vi "Read_Data_file.vi"(0 "Results file":path, 1 "Read Channel Names only":bool, 3 "Add Extra Channels?":bool, 5 "Template File":path, 8 "Desired File Types":T1) -> (10 "Row numbers":i32[](array[numeric]), 11 "Template File Out":path, 12 "Filetype":string, 13 "EOF?":bool, 14 "Results file Out":path, 15 "String Before":string, 16 "Ch names Out":string[](array[string]), 17 "Channel Values Out":string[][](array[string]), 18 "String After":string, 19 "mark after read (chars.)":i32)   [LabVIEW 2010]
uses:
  Data_File_Type.ctl
  Results_plotter_Global.vi
  Globals/Meas_global.vi
panel:
  out "Case":string
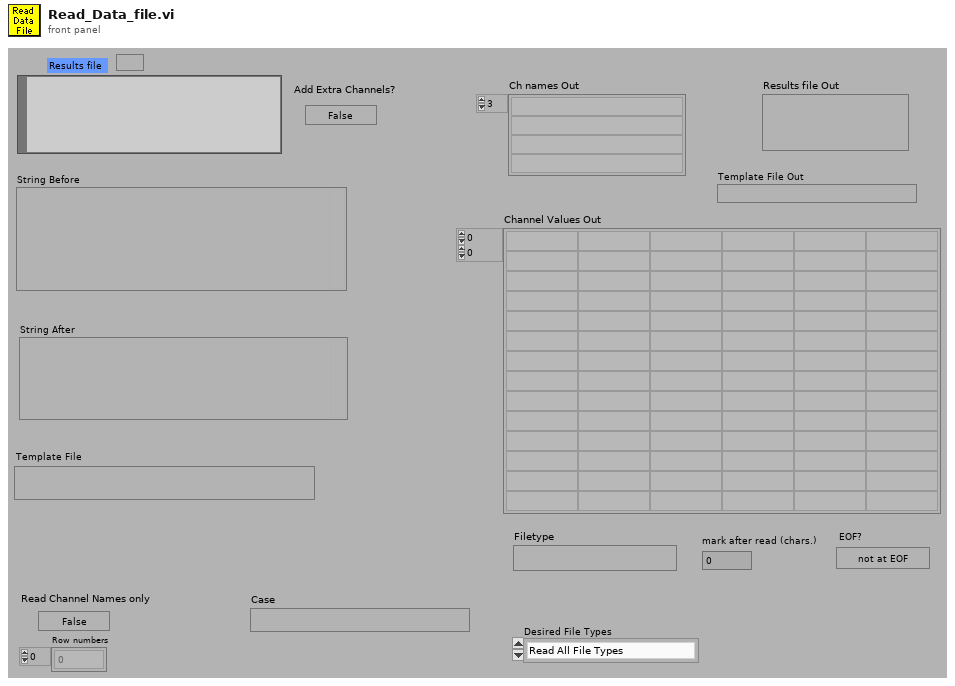
[diagram p1: front panel]
types:
  T1 = typedef "Data_File_Type.ctl" = enum16{"Read All File Types", "Results Files Only", "Raw Data Files Only", "Calibration Files Only", "Gas Desk Files Only", "Old Results Files Only", "Tabulated Data Files Only"}
  T2 = enum32{"existing file", "new file", "new or existing file", "existing dir", "new dir", "new or existing dir", "existing file (use LLBs)", "new file (use LLBs)", "new or existing file (use LLBs)", "new or existing file or directory (use LLBs)"}
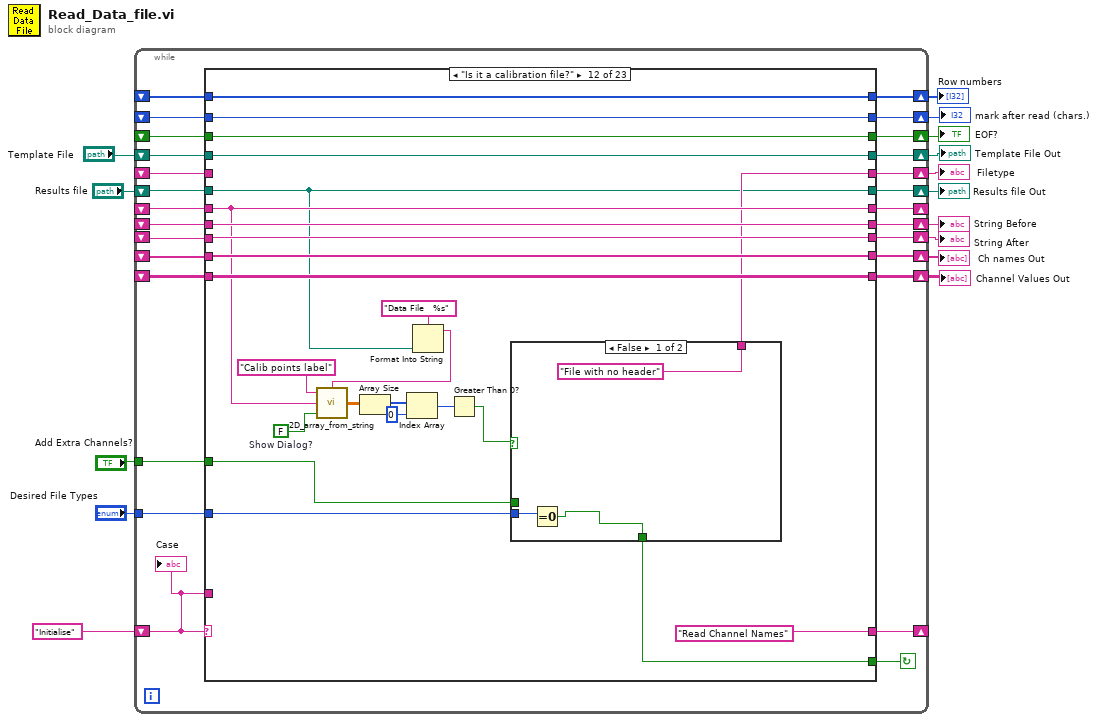
[diagram p0: block diagram]
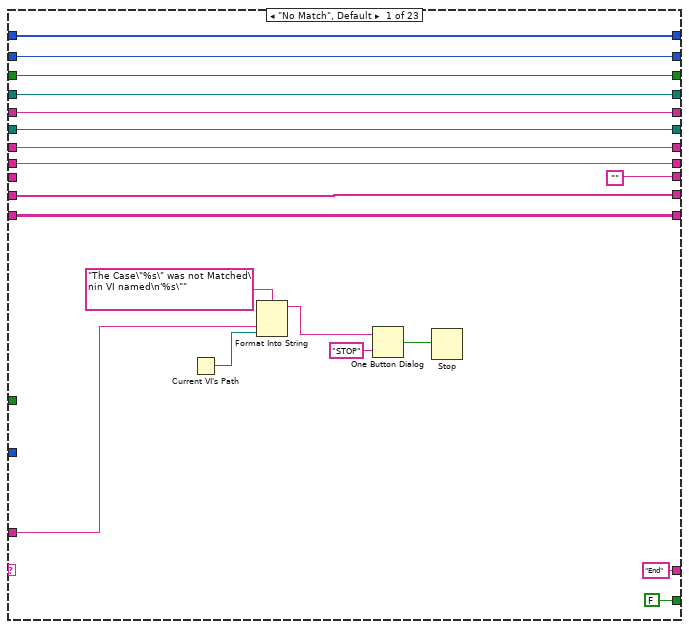
[diagram p2: hidden frame]
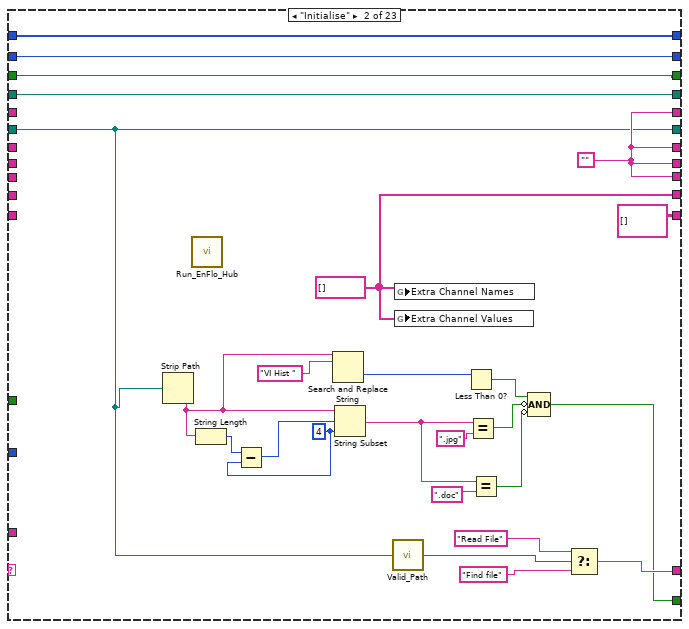
[diagram p3: hidden frame]
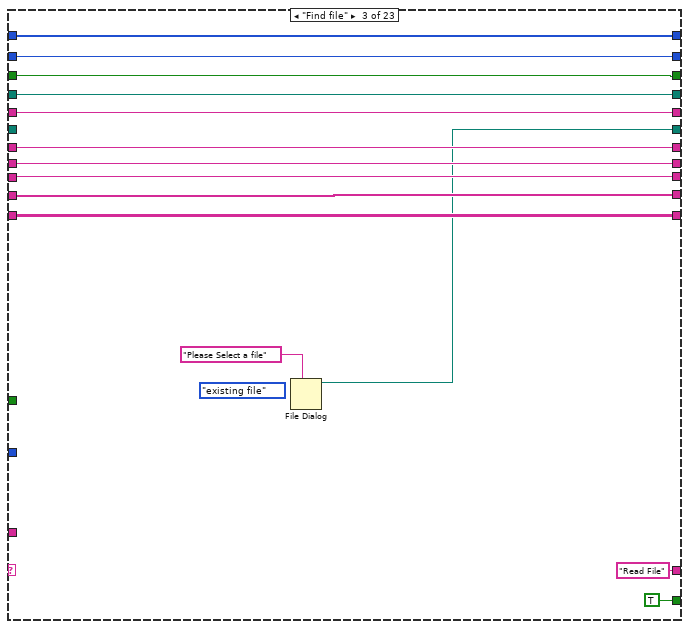
[diagram p4: hidden frame]
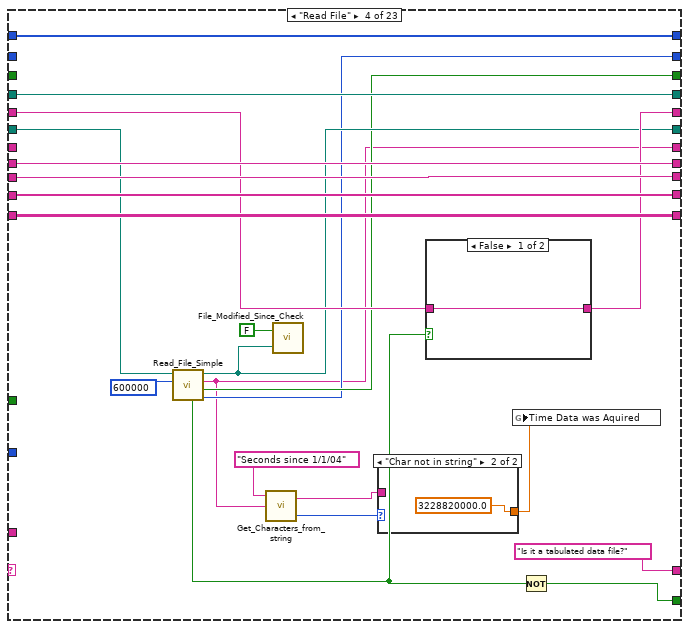
[diagram p5: hidden frame]
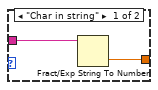
[diagram p6: hidden frame]
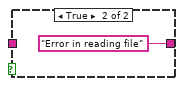
[diagram p7: hidden frame]
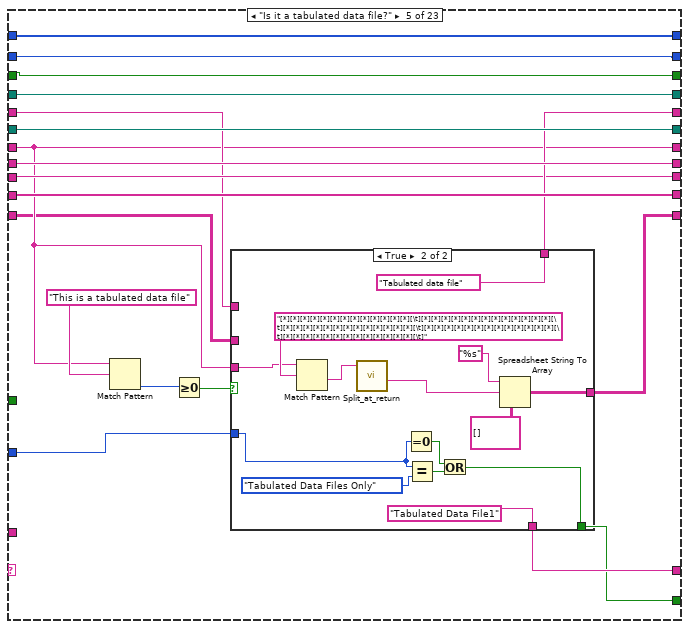
[diagram p8: hidden frame]
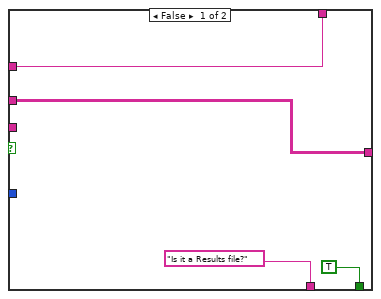
[diagram p9: hidden frame]
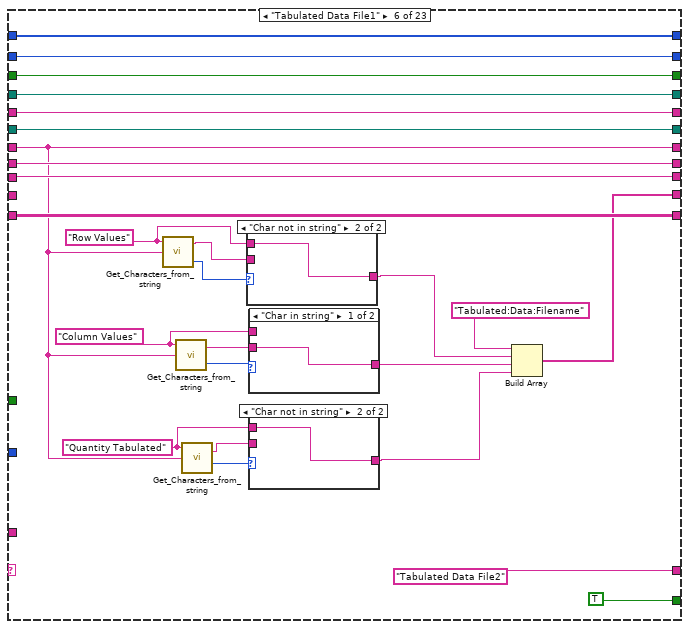
[diagram p10: hidden frame]
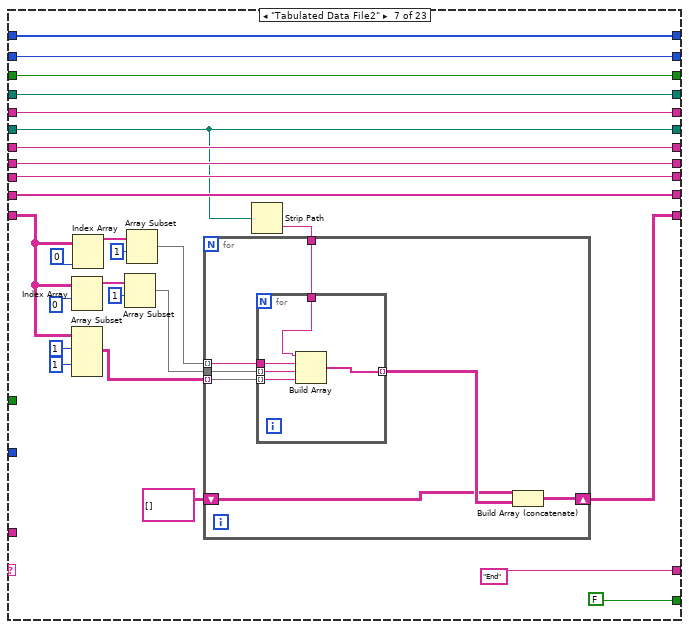
[diagram p14: hidden frame]
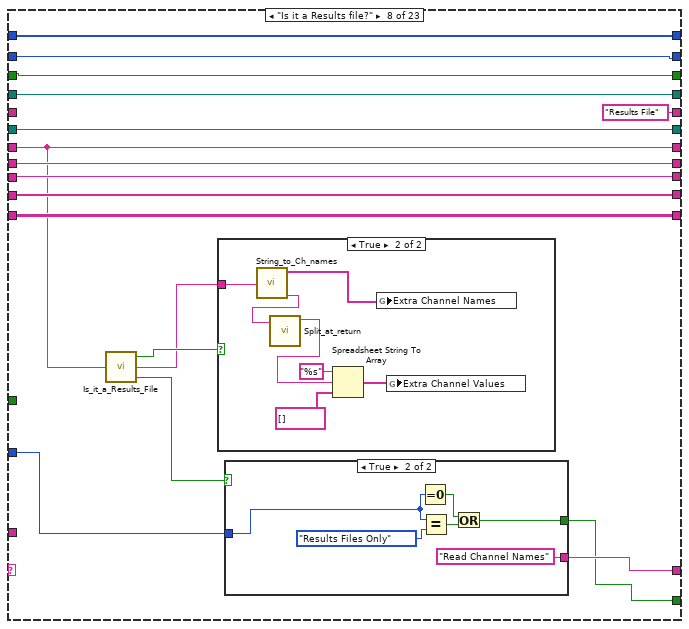
[diagram p15: hidden frame]
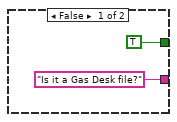
[diagram p16: hidden frame]
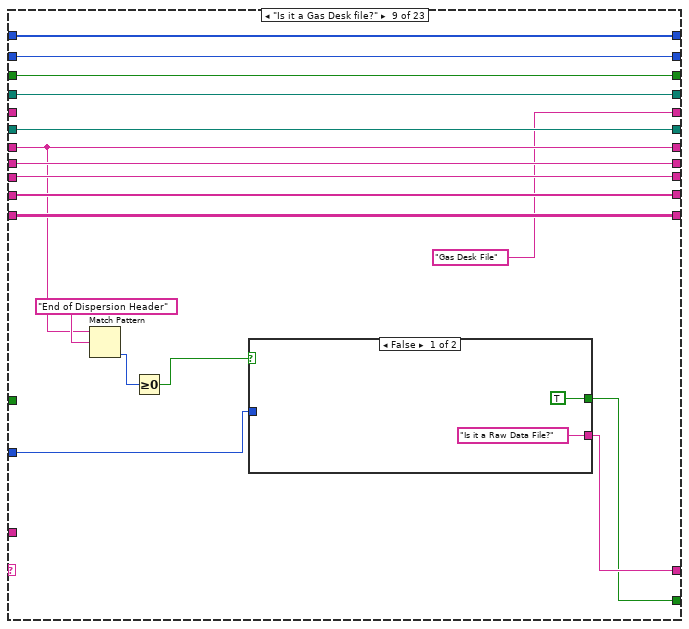
[diagram p18: hidden frame]
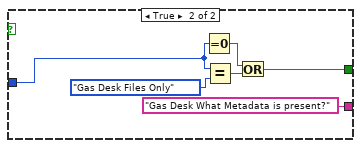
[diagram p19: hidden frame]
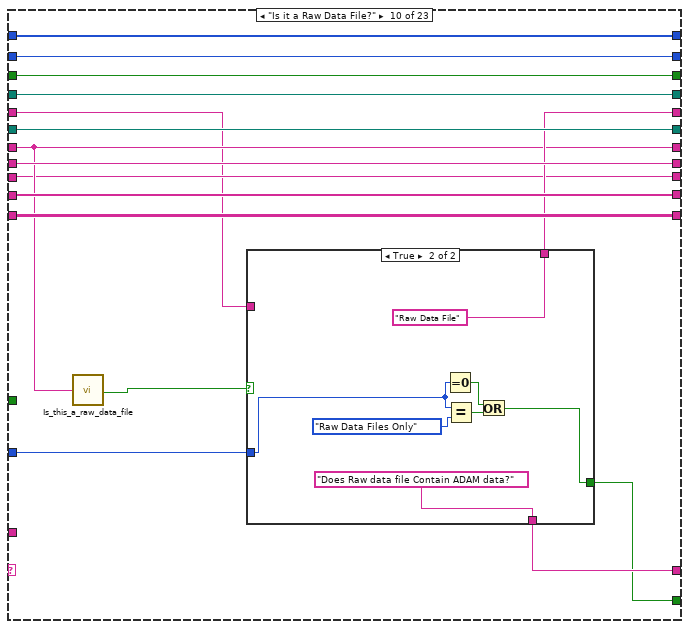
[diagram p20: hidden frame]
diagram:
  n1 = while {
    tunnel: "Add Extra Channels?" -> [w25]
    shift-left: _ -> [w29]
    shift-right: [w28] -> w14
    shift-left: "Results file" -> [w31]
    shift-right: [w30] -> w12
    shift-left: _ -> [w33]
    shift-right: [w32] -> w7
    shift-left: _ -> [w26]
    shift-right: [w34] -> w9
    shift-left: _ -> [w35]
    shift-right: [w36] -> _
    shift-left: "Initialise" -> [w39]
    shift-right: [w37] -> _
    shift-left: _ -> [w27]
    shift-right: [w41] -> w10
    shift-left: _ -> [w38]
    shift-right: [w42] -> w11
    shift-right: [w24] -> w6
    shift-left: "Template File" -> [w23]
    shift-right: [w21] -> w4
    shift-left: _ -> [w22]
    shift-right: [w20] -> w3
    shift-left: _ -> [w19]
    shift-right: [w17] -> w2
    shift-left: _ -> [w18]
    tunnel: "Desired File Types" -> [w16]
    stop <- w40 continue-if-true
    n2 = case shown="\"Is it a calibration file?\"" w39 {
      tunnel: [w54 w85 w99 w121 w146 w172 w223 w252 w284 w308 w336 w370 w404 w425 w464 w492 w505 w567 w590 w626 w652 w684 w703] -> w42
      tunnel: [w53 string[][] [] ("Channel Values") w98 w120 w135 w190 w212 w251 w283 w307 w335 w369 w403 w424 w463 w491 w513 w573 w615 w625 w647 w674 w699] -> w41
      tunnel: [FALSE ("Results File?") w74 TRUE ("Results File?") w117 w128 TRUE ("Results File?") FALSE ("Results File?") w243 w268 w294 w320 w356 w396 TRUE ("Results File?") TRUE ("Results File?") TRUE ("Results File?") w499 TRUE ("Results File?") TRUE ("Results File?") FALSE ("Results File?") TRUE ("Results File?") w678 FALSE ("Results File?")] -> w40
      tunnel: w39 -> [w56 _ _ _ _ _ _ _ _ _ _ _ _ _ _ _ _ _ _ _ _ _ _]
      tunnel: w38 -> [w54 _ w99 w121 w146 _ w223 w252 w284 w308 w336 w370 w404 w425 w464 w492 _ w567 w591 w630 w652 w684 w706]
      tunnel: ["End" w86 "Read File" "Is it a tabulated data file?" w142 "Tabulated Data File2" ("f") "End" ("f") w250 w269 w303 w331 "Read Channel Names" ("f") "Read Channel Names" ("f") w410 "Read Channel Names" ("f") "Read Channel Names" ("f") w503 "Does template file exist?" ("f") w610 "End" ("f") "Delete First Row?" ("f") "Add Extra Channels of data" ("f") "End" ("f")] -> w37
      tunnel: [w51 w83 w96 w103 w136 w183 w219 w245 w277 w301 w326 w365 w392 w412 w442 w475 w506 w568 w614 w631 w645 w686 w708] -> w36
      tunnel: w35 -> [w51 _ w96 _ w136 w183 w219 w245 w277 w301 w326 w365 w399 w411 w442 w475 w508 w568 w614 w631 w645 w686 w708]
      tunnel: [w50 w83 w95 w119 w144 w188 w222 w246 w280 w305 w333 w368 w401 w421 w460 w489 w507 w565 w613 w634 w651 w689 w712] -> w34
      tunnel: w33 -> [_ _ w94 w118 w141 w186 w220 w248 w281 w300 w330 w367 _ w422 w461 w490 w512 w572 w612 w633 w650 w688 w711]
      tunnel: ["" w83 w94 w118 w141 w186 w220 w248 w281 w300 w330 w367 w389 w422 w461 w490 w512 w572 w612 w633 w650 w688 w711] -> w32
      tunnel: w31 -> [w49 w67 _ w114 w145 w189 w202 w249 w282 w306 w334 w348 w402 w423 w462 w469 w511 w571 w608 w629 w644 w685 w707]
      tunnel: [w49 w67 w93 w110 w145 w189 w202 w249 w282 w306 w334 w348 w402 w423 w462 w469 w511 w571 w608 w629 w644 w685 w707] -> w30
      tunnel: w29 -> [w47 _ w91 w115 w140 w185 w218 _ _ w299 w329 _ w395 w409 w458 w487 w510 w570 w611 w628 w641 w683 w710]
      tunnel: [w47 w83 w91 w116 w143 w185 w218 "Results File" "Gas Desk File" w304 w332 w355 w395 w409 w458 w487 w510 w570 w611 w628 w641 w683 w710] -> w28
      tunnel: w27 -> [w53 _ w98 w120 w134 w190 w211 w251 w283 w307 w335 w369 w403 w424 w463 w491 w513 w573 w615 _ _ w682 w701]
      tunnel: w26 -> [w50 _ w95 w119 w144 w188 w222 w246 w280 w305 w333 w368 w401 w421 w460 w489 _ w565 w613 w634 w651 w689 w712]
      tunnel: w25 -> [_ _ _ _ _ _ _ _ _ _ _ w357 _ _ _ _ _ _ _ _ _ w669 _]
      tunnel: [w46 w73 w90 w109 w133 w168 w200 w241 w275 w298 w324 w354 w386 w408 w440 w468 w501 w563 w593 w624 w640 w677 w698] -> w24
      tunnel: w23 -> [w46 w73 w90 w109 w133 w168 w200 w241 w275 w298 w324 w354 w386 w408 w440 w468 w501 w563 w593 w623 w640 w677 w698]
      tunnel: w22 -> [w44 w71 w88 _ w131 w166 w198 w239 w273 w296 w322 w352 w384 w406 w438 w466 w500 w562 w602 w622 w639 w675 w696]
      tunnel: [w44 w71 w88 w108 w131 w166 w198 w239 w273 w296 w322 w352 w384 w406 w438 w466 w500 w562 w602 w622 w638 w675 w696] -> w21
      tunnel: [w45 w72 w89 w107 w132 w167 w199 w240 w274 w297 w323 w353 w385 w407 w439 w467 w496 w561 w601 w621 w637 w676 w697] -> w20
      tunnel: w19 -> [w45 w72 w89 _ w132 w167 w199 w240 w274 w297 w323 w353 w385 w407 w439 w467 w497 w561 w601 w621 w637 w676 w697]
      tunnel: [w43 w70 w87 w106 w130 w165 w197 w238 w272 w295 w321 w351 w383 w405 w437 w465 w493 w560 w600 w620 w636 w670 w695] -> w17
      tunnel: w18 -> [w43 w70 w87 w106 w130 w165 w197 w238 w272 w295 w321 w351 w383 w405 w437 w465 w493 w560 w600 _ w636 _ w695]
      tunnel: w16 -> [_ _ _ _ w129 _ _ w236 w271 w293 w319 w350 _ _ _ _ _ _ _ _ _ _ _]
      frame "No Match", Default {
        n3 = Current VI's Path() -> (path=w57:path)
        n4 = Format Into String(format string="The Case\"%s\" was not Matched\nin VI named\n'%s\"" ("Format String"), w56, w57) -> (resulting string=w60:string)  [unwired: 2 in, 1 out]
        n5 = One Button Dialog(message=w60, button name ("OK")="STOP") -> (true=w58:bool)
        n6 = Stop(stop? (T)=w58) -> ()
      }
      frame "Initialise" {
        w81 = 4 ("length (rest)")
        w83 = ""
        w85 = string[] [] ("Extra Channel Names")
        n7 = Strip Path(path=w67) -> (name=w79:string)  [unwired: 1 out]
        n8 = call "Run_EnFlo_Hub.vi"() -> ()  [unwired: 8 out]
        n9 = String Length(string=w79) -> (length=w82:i32)
        n10 = Subtract(x=w82, y=w81) -> (x-y=w80:i32)
        n11 = Search and Replace String(input string=w79, search string="VI Hist ") -> (offset past replacement=w77:i32)  [unwired: 1 in, 8 out]
        n12 = String Subset(string=w79, offset (0)=w80, length (rest)=w81) -> (substring=w64:string)
        n13 = call "Valid_Path.vi"("Filename"=w67) -> ("Valid Path?"=w66:bool)
        n14 = global write "Results_plotter_Global.vi" "Extra Channel Names"(w85) -> ()
        n15 = global write "Results_plotter_Global.vi" "Extra Channel Values"(w85) -> ()
        n16 = Less Than 0?(x=w77) -> (x < 0?=w75:bool)
        n17 = Equal?(x=w64, y=".jpg") -> (x = y?=w76:bool)
        n18 = Equal?(x=w64, y=".doc") -> (x = y?=w63:bool)
        n19 = Compound Arithmetic op=AND(w75, invert w76, invert w63) -> (w74:bool)
        n20 = Select(t="Read File", s=w66, f="Find file") -> (s? t:f=w86:string)
      }
      frame "Find file" {
        (unwired) T2."existing file" ("select mode (2)")
        n21 = File Dialog(7:"Please Select a file" ("prompt")) -> (3:w93:path)  [unwired: 1 in, 8 out]
      }
      frame "Read File" {
        n22 = call "Read_File_Simple.vi"("Filename"=w114, "number of characters (all:-1)"=600000 ("count")) -> ("Error?"=w112:bool, "Filename Out"=w110:path, "string"=w103:string, "EOF?"=w108:bool, "mark after read (chars.)"=w107:i32)  [unwired: 1 in, 3 out]
        n23 = call "Get_Characters_from_string.vi"("Input string"=w103, "Variable name"="Seconds since 1/1/04") -> ("Status"=w101:enum16{"Char in string", "Char not in string"}, "Value"=w104:string)  [unwired: 1 in]
        n24 = call "File_Modified_Since_Check.vi"("Pathname"=w110, "Just Modified?"=FALSE) -> ()  [unwired: 1 out]
        n25 = case shown="\"Char not in string\"" w101 {
          tunnel: w104 -> [w124 _]
          tunnel: [w123 3228820000.0 ("y")] -> w102
          frame "Char in string" {
            n26 = Fract/Exp String To Number(string=w124) -> (number=w123:dbl)  [unwired: 4 out]
          }
          frame "Char not in string" {
          }
        }
        n27 = case shown="False" w112 {
          tunnel: [w126 "Error in reading file"] -> w116
          tunnel: w115 -> [w126 _]
          frame False {
          }
          frame True {
          }
        }
        n28 = global write "Meas_global.vi" "Time Data was Aquired"(w102) -> ()
        n29 = Not(x=w112) -> (.not. x?=w117:bool)
      }
      frame "Is it a tabulated data file?" {
        n30 = Match Pattern(string=w136, regular expression="This is a tabulated data file") -> (offset past match=w139:i32)  [unwired: 4 out]
        n31 = Greater Or Equal To 0?(x=w139) -> (x >= 0?=w138:bool)
        n32 = case shown="True" w138 {
          tunnel: [w150 "Tabulated data file"] -> w143
          tunnel: ["Is it a Results file?" "Tabulated Data File1" ("f")] -> w142
          tunnel: w140 -> [w150 _]
          tunnel: w136 -> [_ w161]
          tunnel: [w149 w158] -> w135
          tunnel: w134 -> [w149 _]
          tunnel: w129 -> [_ w154]
          tunnel: [TRUE ("Results File?") w151] -> w128
          frame False {
          }
          frame True {
            n33 = Match Pattern(string=w161, regular expression="[*][*][*][*][*][*][*][*][*][*][*][*][*][\t][*][*][*][*][*][*][*][*][*][*][*][*][*][\t][*][*][*][*][*][*][*][*][*][*][*][*][*][\t][*][*][*][*][*][*][*][*][*][*][*][*][*][\t][*][*][*][*][*][*][*][*][*][*][*][*][*][\t]" ("String")) -> (after substring=w157:string)  [unwired: 4 out]
            n34 = call "Split_at_return.vi"("String"=w157) -> ("after substring"=w156:string)  [unwired: 1 in, 3 out]
            n35 = Equal To 0?(x=w154) -> (x = 0?=w152:bool)
            n36 = Equal?(x=w154, y=Data_File_Type."Tabulated Data Files Only" ("Desired File Types")) -> (x = y?=w153:bool)
            n37 = Or(x=w152, y=w153) -> (x .or. y?=w151:bool)
            n38 = Spreadsheet String To Array(format string="%s", spreadsheet string=w156, array type (2D Dbl)=string[][] [] ("Channel Values")) -> (array=w158:string[][])  [unwired: 1 out]
          }
        }
      }
      frame "Tabulated Data File1" {
        w171 = "Row Values" ("Variable name")
        w170 = "Column Values" ("Variable name")
        w177 = "Quantity Tabulated" ("Variable name")
        n39 = call "Get_Characters_from_string.vi"("Input string"=w183, "Variable name"=w171) -> ("Status"=w175:enum16{"Char in string", "Char not in string"}, "Value"=w176:string)  [unwired: 1 in]
        n40 = call "Get_Characters_from_string.vi"("Input string"=w183, "Variable name"=w170) -> ("Status"=w182:enum16{"Char in string", "Char not in string"}, "Value"=w181:string)  [unwired: 1 in]
        n41 = call "Get_Characters_from_string.vi"("Input string"=w183, "Variable name"=w177) -> ("Status"=w179:enum16{"Char in string", "Char not in string"}, "Value"=w178:string)  [unwired: 1 in]
        n42 = case shown="\"Char not in string\"" w175 {
          tunnel: w176 -> [w193 _]
          tunnel: [w193 w194] -> w174
          tunnel: w171 -> [_ w194]
          frame "Char in string" {
          }
          frame "Char not in string" {
          }
        }
        n43 = case shown="\"Char in string\"" w182 {
          tunnel: w181 -> [w195 _]
          tunnel: [w195 w196] -> w180
          tunnel: w170 -> [_ w196]
          frame "Char in string" {
          }
          frame "Char not in string" {
          }
        }
        n44 = case shown="\"Char not in string\"" w179 {
          tunnel: w178 -> [w191 _]
          tunnel: [w191 w192] -> w173
          tunnel: w177 -> [_ w192]
          frame "Char in string" {
          }
          frame "Char not in string" {
          }
        }
        n45 = Build Array("Tabulated:Data:Filename", w174, w180, w173) -> (w172:string[])
      }
      frame "Tabulated Data File2" {
        n46 = Index Array(array=w211, index (row)=0) -> (element=w210:string[])  [unwired: 1 in]
        n47 = Array Subset(array=w211, index (row)=1 ("index"), index (col)=1 ("index")) -> (w214:string[][])  [unwired: 2 in]
        n48 = Index Array(array=w211, index (col)=0 ("index (row)")) -> (element=w206:string[])  [unwired: 1 in]
        n49 = Array Subset(array=w210, index=1) -> (w207:string[])  [unwired: 1 in]
        n50 = Array Subset(array=w206, index=1) -> (w205:string[])  [unwired: 1 in]
        n51 = Strip Path(path=w202) -> (name=w201:string)  [unwired: 1 out]
        n52 = for {
          tunnel: w205 -> [w230] mode=indexing
          tunnel: w207 -> [w229]
          tunnel: w214 -> [w228] mode=indexing
          shift-right: [w225] -> w212
          shift-left: string[][] [] -> [w226]
          tunnel: w201 -> [w224]
          n53 = for {
            tunnel: w230 -> [w235]
            tunnel: w229 -> [w234] mode=indexing
            tunnel: w228 -> [w233] mode=indexing
            tunnel: [w232] -> w227 mode=indexing
            tunnel: w224 -> [w231]
            n54 = Build Array(w231, w235, w234, w233) -> (w232:string[])
          }
          n55 = Build Array (concatenate)(w226, w227) -> (w225:string[][])
        }
      }
      frame "Is it a Results file?" {
        n56 = call "Is_it_a_Results_File.vi"("character string"=w245) -> ("Contain DB Header Info"=w244:bool, "Header String"=w237:string, "Results File?"=w242:bool)
        n57 = case shown="True" w244 {
          tunnel: w237 -> [_ w263]
          frame False {
          }
          frame True {
            n58 = call "String_to_Ch_names.vi"("Spreadsheet string"=w263) -> ("Ch names"=w262:string[], "String After names"=w266:string)  [unwired: 2 out]
            n59 = call "Split_at_return.vi"("String"=w266) -> ("before substring"=w267:string)  [unwired: 1 in, 3 out]
            n60 = Spreadsheet String To Array(format string="%s", spreadsheet string=w267, array type (2D Dbl)=string[] [] ("Channel Values")) -> (array=w261:string[])  [unwired: 1 out]
            n61 = global write "Results_plotter_Global.vi" "Extra Channel Names"(w262) -> ()
            n62 = global write "Results_plotter_Global.vi" "Extra Channel Values"(w261) -> ()
          }
        }
        n63 = case shown="True" w242 {
          tunnel: ["Is it a Gas Desk file?" "Read Channel Names"] -> w250
          tunnel: w236 -> [_ w257]
          tunnel: [TRUE w255] -> w243
          frame False {
          }
          frame True {
            n64 = Equal To 0?(x=w257) -> (x = 0?=w258:bool)
            n65 = Equal?(x=w257, y=Data_File_Type."Results Files Only" ("Desired File Types")) -> (x = y?=w259:bool)
            n66 = Or(x=w258, y=w259) -> (x .or. y?=w255:bool)
          }
        }
      }
      frame "Is it a Gas Desk file?" {
        n67 = Match Pattern(string=w277, regular expression="End of Dispersion Header") -> (offset past match=w279:i32)  [unwired: 4 out]
        n68 = Greater Or Equal To 0?(x=w279) -> (x >= 0?=w270:bool)
        n69 = case shown="False" w270 {
          tunnel: ["Is it a Raw Data File?" "Gas Desk What Metadata is present?"] -> w269
          tunnel: w271 -> [_ w289]
          tunnel: [TRUE w287] -> w268
          frame False {
          }
          frame True {
            n70 = Equal To 0?(x=w289) -> (x = 0?=w290:bool)
            n71 = Equal?(x=w289, y=Data_File_Type."Gas Desk Files Only" ("Desired File Types")) -> (x = y?=w291:bool)
            n72 = Or(x=w290, y=w291) -> (x .or. y?=w287:bool)
          }
        }
      }
      frame "Is it a Raw Data File?" {
        n73 = call "Is_this_a_raw_data_file.vi"("character string"=w301) -> ("Raw Dat File?"=w302:bool)  [unwired: 2 out]
        n74 = case shown="True" w302 {
          tunnel: [w310 "Raw Data File"] -> w304
          tunnel: ["Is it an older results file?" ("f") "Does Raw data file Contain ADAM data?" ("f")] -> w303
          tunnel: w299 -> [w310 _]
          tunnel: [TRUE ("Results File?") w313] -> w294
          tunnel: w293 -> [_ w314]
          frame False {
          }
          frame True {
            n75 = Equal To 0?(x=w314) -> (x = 0?=w316:bool)
            n76 = Equal?(x=w314, y=Data_File_Type."Raw Data Files Only" ("Desired File Types")) -> (x = y?=w315:bool)
            n77 = Or(x=w316, y=w315) -> (x .or. y?=w313:bool)
          }
        }
      }
      frame "Is it an older results file?" {
        n78 = Match Pattern(string=w326, regular expression="Date of meas\tTime of meas") -> (offset past match=w327:i32)  [unwired: 4 out]
        n79 = Greater Or Equal To 0?(x=w327) -> (x >= 0?=w325:bool)
        n80 = case shown="True" w325 {
          tunnel: [w339 "Older Results File"] -> w332
          tunnel: ["Is it a calibration file?" ("f") "Read Channel Names" ("f")] -> w331
          tunnel: w329 -> [w339 _]
          tunnel: [TRUE ("Results File?") w341] -> w320
          tunnel: w319 -> [_ w340]
          frame False {
          }
          frame True {
            n81 = Equal To 0?(x=w340) -> (x = 0?=w344:bool)
            n82 = Equal?(x=w340, y=Data_File_Type."Old Results Files Only" ("Desired File Types")) -> (x = y?=w343:bool)
            n83 = Or(x=w344, y=w343) -> (x .or. y?=w341:bool)
          }
        }
      }
      frame "Is it a calibration file?" {
        w364 = FALSE  # Show Dialog?
        n84 = Format Into String(format string="Data File   %s", w348) -> (resulting string=w347:string)  [unwired: 2 in, 1 out]
        n85 = call "2D_array_from_string.vi"("String Name"=w347, "Show Dialog?"=w364, "Input string"=w365, "Array title"="Calib points label") -> ("2D data array"=w363:dbl[][])
        n86 = Array Size(array=w363) -> (size(s)=w362:i32[])
        n87 = Index Array(array=w362, index=0 ("Index")) -> (element=w360:i32)
        n88 = Greater Than 0?(x=w360) -> (x > 0?=w358:bool)
        n89 = case shown="False" w358 {
          tunnel: w357 -> [_ w382]
          tunnel: [w371 w374] -> w356
          tunnel: ["File with no header" "Calibration File"] -> w355
          tunnel: w350 -> [w372 w378]
          frame False {
            n90 = Equal To 0?(x=w372) -> (x = 0?=w371:bool)
          }
          frame True {
            n91 = Not(x=w382) -> (.not. x?=w375:bool)
            n92 = Equal To 0?(x=w378) -> (x = 0?=w380:bool)
            n93 = Equal?(x=w378, y=Data_File_Type."Calibration Files Only" ("Desired File Types")) -> (x = y?=w379:bool)
            n94 = Or(x=w380, y=w379) -> (x .or. y?=w376:bool)
            n95 = Or(x=w376, y=w375) -> (x .or. y?=w374:bool)
          }
        }
      }
      frame "Does Raw data file Contain ADAM data?" {
        w387 = "\r"
        w390 = "Raw data header Start"
        n96 = Match Pattern(string=w399, regular expression=w390) -> (before substring=w393:string, after substring=w388:string)  [unwired: 3 out]
        n97 = Match Pattern(string=w393, regular expression="[*][*][*][*][*][*][*][*][*][*][*][*][*][*][*][*][*][*][*][*][*]" ("String")) -> (before substring=w392:string)  [unwired: 4 out]
        n98 = Concatenate Strings(w387, "************************", w387, w390, w388) -> (w389:string)
        n99 = String Length(string=w393) -> (length=w398:i32)
        n100 = Greater?(x=w398, y=30) -> (0:w396:bool)
      }
      frame "Gas Desk What Metadata is present?" {
        n101 = String Subset(string=w411, offset (0)=0, length (rest)=6 ("length")) -> (substring=w418:string)
        n102 = Equal?(x="******", y=w418) -> (x = y?=w416:bool)
        n103 = case shown="False" w416 {
          tunnel: [w427 "Gas Desk Read ADAM ch's Header"] -> w410
          tunnel: w411 -> [w426 _]
          frame False {
            w431 = "Data Base\tData Base\tData Base\t"
            n104 = String Length(string=w431) -> (length=w434:i32)
            n105 = String Subset(string=w426, offset (0)=0, length (rest)=w434) -> (substring=w432:string)
            n106 = Equal?(x=w431, y=w432) -> (x = y?=w430:bool)
            n107 = Select(t="Gas Desk DB Header Present", s=w430, f="Read Channel Names") -> (s? t:f=w427:string)
          }
          frame True {
          }
        }
        n108 = call "Fast_string_Replace.vi"("Replace match with:"="Suspect Pulse Width" ("regular expression"), "Input String"=w411, "regular expression"="Suspect \u0003Pulse Width ") -> ("Output String"=w412:string)  [unwired: 2 out]
      }
      frame "Gas Desk DB Header Present" {
        w445 = string[] [] ("Channel Values")
        n109 = call "String_to_Ch_names.vi"("Spreadsheet string"=w442) -> ("Ch names"=w457:string[], "String After names"=w446:string)  [unwired: 2 out]
        n110 = call "Split_at_return.vi"("String"=w446) -> ("before substring"=w448:string, "after substring"=w449:string)  [unwired: 1 in, 2 out]
        n111 = call "Split_at_return.vi"("String"=w449) -> ("after substring"=w450:string)  [unwired: 1 in, 3 out]
        n112 = call "String_to_Ch_names.vi"("Spreadsheet string"=w450) -> ("Ch names"=w456:string[], "String After names"=w451:string)  [unwired: 2 out]
        n113 = call "Split_at_return.vi"("String"=w451) -> ("after substring"=w453:string)  [unwired: 1 in, 3 out]
        n114 = call "Split_at_return.vi"("String"=w453) -> ("before substring"=w454:string)  [unwired: 1 in, 3 out]
        n115 = Spreadsheet String To Array(format string="%s", spreadsheet string=w448, array type (2D Dbl)=w445) -> (array=w444:string[])  [unwired: 1 out]
        n116 = Spreadsheet String To Array(format string="%s", spreadsheet string=w454, array type (2D Dbl)=w445) -> (array=w455:string[])  [unwired: 1 out]
        n117 = Build Array (concatenate)(w456, w457) -> (w436:string[])
        n118 = Build Array (concatenate)(w455, w444) -> (w443:string[])
        n119 = global write "Results_plotter_Global.vi" "Extra Channel Values"(w443) -> ()
        n120 = global write "Results_plotter_Global.vi" "Extra Channel Names"(w436) -> ()
      }
      frame "Gas Desk Read ADAM ch's Header" {
        n121 = call "Split_at_return.vi"("String"=w475) -> ("after substring"=w483:string)  [unwired: 1 in, 3 out]
        n122 = call "String_to_Ch_names.vi"("Spreadsheet string"=w483) -> ("Ch names"=w471:string[], "String After names"=w484:string)  [unwired: 2 out]
        n123 = call "Split_at_return.vi"("String"=w484) -> ("after substring"=w485:string)  [unwired: 1 in, 3 out]
        n124 = call "Split_at_return.vi"("String"=w485) -> ("before substring"=w482:string)  [unwired: 1 in, 3 out]
        n125 = Spreadsheet String To Array(format string="%s", spreadsheet string=w482, array type (2D Dbl)=string[] [] ("Channel Values")) -> (array=w476:string[])  [unwired: 1 out]
        n126 = Strip Path(path=w469) -> (stripped path=w478:path, name=w477:string)
        n127 = Path To String(path=w478) -> (string=w479:string)
        n128 = Build Array (concatenate)("Original:Results:Filename", "Original:Results:Filepath", w471) -> (w470:string[])
        n129 = Build Array (concatenate)(w477, w479, w476) -> (w474:string[])
        n130 = global write "Results_plotter_Global.vi" "Extra Channel Names"(w470) -> ()
        n131 = global write "Results_plotter_Global.vi" "Extra Channel Values"(w474) -> ()
      }
      frame "Read Channel Names" {
        n132 = case shown="\"Older Results File\"" w510 {
          tunnel: [w521 w535 w544 0 0] -> w494
          tunnel: [w520 w534 w548 w553 w558] -> w504
          tunnel: w508 -> [w519 w536 w547 w556 w558]
          tunnel: [w518 w542 "Is Raw Data Filename Present?" ("f") w551 w557] -> w503
          tunnel: "Does template file exist?" ("f") -> [w518 w542 _ w551 w557]
          frame "Results File" {
            n133 = Match Pattern(string=w519, regular expression="[*][*][*][*][*][*][*][*][*][*][*][*][*][\t][*][*][*][*][*][*][*][*][*][*][*][*][*][\t][*][*][*][*][*][*][*][*][*][*][*][*][*][\t][*][*][*][*][*][*][*][*][*][*][*][*][*][\t][*][*][*][*][*][*][*][*][*][*][*][*][*][\t]" ("String")) -> (after substring=w524:string, offset past match=w522:i32)  [unwired: 3 out]
            n134 = call "Split_at_return.vi"("String"=w524) -> ("after substring"=w520:string, "offset past match"=w523:i32)  [unwired: 1 in, 2 out]
            n135 = Add(x=w522, y=w523) -> (x+y=w521:i32)
          }
          frame "Older Results File" {
            w529 = "\r"
            n136 = Match Pattern(string=w536, regular expression="Date of meas\tTime of meas") -> (before substring=w540:string, match substring=w533:string, offset past match=w537:i32)  [unwired: 2 out]
            n137 = Reverse String(1:w540) -> (0:w539:string)
            n138 = String Length(string=w533) -> (length=w532:i32)
            n139 = Match Pattern(string=w539, regular expression=w529) -> (after substring=w538:string, offset past match=w530:i32)  [unwired: 3 out]
            n140 = Match Pattern(string=w538, regular expression=w529) -> (after substring=w528:string, offset past match=w531:i32)  [unwired: 3 out]
            n141 = Match Pattern(string=w528, regular expression=w529) -> (offset past match=w527:i32)  [unwired: 4 out]
            n142 = Compound Arithmetic op=ADD(invert w532, w537, invert w531, invert w530, invert w527, 1 ("value")) -> (w535:i32)
            n143 = Search/Split String(string=w536, offset (0)=w535) -> (match + rest of string=w534:string)  [unwired: 3 out]
          }
          frame "Gas Desk File" {
            n144 = Match Pattern(string=w547, regular expression="End of Dispersion Header") -> (after substring=w550:string, offset past match=w545:i32)  [unwired: 3 out]
            n145 = call "Split_at_return.vi"("String"=w550) -> ("after substring"=w548:string, "offset past match"=w546:i32)  [unwired: 1 in, 2 out]
            n146 = Add(x=w546, y=w545) -> (x+y=w544:i32)
          }
          frame "Raw Data File" {
            n147 = Search/Split String(string=w556, offset (0)=37 ("y")) -> (match + rest of string=w555:string)  [unwired: 3 out]
            n148 = call "Split_at_return.vi"("String"=w555) -> ("after substring"=w553:string)  [unwired: 1 in, 3 out]
          }
          frame "File with no header", Default {
          }
        }
        n149 = call "String_to_Ch_names.vi"("Spreadsheet string"=w504) -> ("Ch names"=w505:string[], "Title length (Bytes)"=w495:i32, "String After names"=w506:string)  [unwired: 1 out]
        n150 = case shown="True" "Read Channel Names only" {
          tunnel: w497 -> [w514 _]
          tunnel: [w514 w515] -> w496
          tunnel: w495 -> [_ w517]
          tunnel: w494 -> [_ w516]
          frame False {
          }
          frame True {
            n151 = Add(x=w516, y=w517) -> (x+y=w515:i32)
          }
        }
        n152 = String Subset(string=w508, offset (0)=0, length (rest)=w494) -> (substring=w507:string)
        n153 = Not(x="Read Channel Names only") -> (.not. x?=w499:bool)
      }
      frame "Is Raw Data Filename Present?" {
        w564 = "Raw:Data:Filename"
        n154 = Search 1D Array(1D array=w567, element=w564) -> (index of element=w566:i32)  [unwired: 1 out]
        n155 = case shown="-1" w566 {
          tunnel: w565 -> [_ w587]
          tunnel: w564 -> [_ w581]
          frame 0, Default {
          }
          frame -1 {
            n156 = global read "Results_plotter_Global.vi" "Extra Channel Names"() -> (w582:string[])
            n157 = global read "Results_plotter_Global.vi" "Extra Channel Values"() -> (w580:string[])
            n158 = Concatenate Strings("Raw data Directory", "\t") -> (w584:string)
            n159 = Match Pattern(string=w587, regular expression=w584) -> (after substring=w583:string)  [unwired: 4 out]
            n160 = call "Split_at_return.vi"("String"=w583) -> ("before substring"=w576:string)  [unwired: 1 in, 3 out]
            n161 = Build Array (concatenate)(w582, w581) -> (w578:string[])
            n162 = global write "Results_plotter_Global.vi" "Extra Channel Names"(w578) -> ()
            n163 = Match Pattern(string=w576, regular expression="\t") -> (before substring=w575:string)  [unwired: 4 out]
            n164 = Build Array (concatenate)(w580, w575) -> (w579:string[])
            n165 = global write "Results_plotter_Global.vi" "Extra Channel Values"(w579) -> ()
          }
        }
      }
      frame "Does template file exist?" {
        n166 = global read "Results_plotter_Global.vi" "Extra Channel Names"() -> (w609:string[])
        n167 = while {
          shift-right: [w618] -> w597
          shift-left: _ -> [w619]
          stop <- TRUE stop-if-true
          n168 = Increment(x=w619) -> (x+1=w618:dbl)
        }
        n169 = call "Common_Extra_Chs.vi"() -> ("Common Extra Channels"=w599:string[])
        n170 = call "Valid_Path.vi"("Filename"=w593) -> ("Valid Path?"=w592:bool)
        n171 = Path to Array of Strings(0:w608) -> (2:w607:string[])  [unwired: 1 out]
        n172 = global read "Results_plotter_Global.vi" "Extra Channel Values"() -> (w605:string[])
        n173 = Build Array (concatenate)(w609, w599) -> (w589:string[])
        n174 = Reverse 1D Array(array=w607) -> (reversed array=w606:string[])
        n175 = call "Update_Ch_Names.vi"("Ch Name in"=w589) -> ("Ch Name Out"=w588:string[])
        n176 = Array Subset(array=w606, length=5) -> (w604:string[])  [unwired: 1 in]
        n177 = Number To Decimal String(number=w597) -> (decimal integer string=w596:string)  [unwired: 1 out]
        n178 = Select(t="Read Values using Template", s=w592, f="Entire string to 2D array") -> (s? t:f=w610:string)
        n179 = Build Array (concatenate)(w605, w604, w596) -> (w603:string[])
        n180 = global write "Results_plotter_Global.vi" "Extra Channel Names"(w588) -> ()
        n181 = call "Update_Ch_Names.vi"("Ch Name in"=w591) -> ("Ch Name Out"=w590:string[])
        n182 = global write "Results_plotter_Global.vi" "Extra Channel Values"(w603) -> ()
      }
      frame "Read Values using Template" {
        n183 = call "Filter_on_template_file_new.vi"("Filetype"=w628, "Filename"=w629, "End Of File already Reached?"=w622, "Start of data (bytes)"=w621, "Data string"=w631, "Channel Names In"=w630, "Template File"=w623) -> ("Data Out"=w627:string[][], "Channel Names Out"=w626:string[], "Row numbers"=w620:i32[], "Template File-write"=w624:path)  [unwired: 1 out]
        n184 = call "Surface_modularity.vi"("Data in"=w627, "Channel names"=w626) -> ("Data out"=w625:string[][])  [unwired: 1 out]
      }
      frame "Entire string to 2D array" {
        n185 = case shown="\"False\", Default" w641 {
          tunnel: [w658 w668] -> w646
          tunnel: w645 -> [w657 w668]
          tunnel: w644 -> [w656 _]
          tunnel: w639 -> [w654 w667]
          tunnel: [w655 w667] -> w638
          tunnel: w637 -> [w653 _]
          frame "False", Default {
            n186 = case shown="False" w654 {
              tunnel: [w662 w666] -> w658
              tunnel: w657 -> [w664 w666]
              tunnel: w656 -> [w661 _]
              tunnel: [w660 w665] -> w655
              tunnel: w654 -> [_ w665]
              tunnel: w653 -> [w659 _]
              frame False {
                n187 = call "Read_Characters_From_File.ph.vi"("file path (dialog if empty)"=w661, "start of read offset (chars.: 0)"=w659) -> ("character string"=w663:string, "EOF?"=w660:bool)  [unwired: 1 in, 5 out]
                n188 = Concatenate Strings(w664, w663) -> (w662:string)
              }
              frame True {
              }
            }
          }
          frame "Raw Data File" {
          }
        }
        n189 = Spreadsheet String To Array(format string="%s", spreadsheet string=w646, array type (2D Dbl)=string[][] [] ("Channel Values")) -> (array=w647:string[][])  [unwired: 1 out]
      }
      frame "Delete First Row?" {
        n190 = global read "Results_plotter_Global.vi" "Extra Channel Names"() -> (w681:string[])
        n191 = case shown="True" w669 {
          tunnel: w683 -> [_ w694]
          tunnel: w682 -> [w691 w693]
          tunnel: [w691 w692] -> w674
          frame False {
          }
          frame True {
            n192 = call "Delete_First_Rows.vi"("Data In"=w693, "File Type"=w694) -> ("Data Out"=w692:string[][])  [unwired: 1 out]
          }
        }
        n193 = Array Size(array=w681) -> (size(s)=w680:i32)
        n194 = Greater Than 0?(x=w680) -> (x > 0?=w679:bool)
        n195 = And(x=w669, y=w679) -> (x .and. y?=w678:bool)
        n196 = Array Size(array=w674) -> (size(s)=w673:i32[])
        n197 = Index Array(array=w673, index=0) -> (element=w671:i32)
        n198 = for {
          N: w671 -> [_]
          tunnel: [w690] -> w670 mode=indexing
          i -> [w690]
        }
      }
      frame "Add Extra Channels of data" {
        n199 = global read "Results_plotter_Global.vi" "Extra Channel Names"() -> (w704:string[])
        n200 = global read "Results_plotter_Global.vi" "Extra Channel Values"() -> (w702:string[])
        n201 = for {
          tunnel: w704 -> [w721] mode=indexing
          shift-right: [w719] -> w700
          shift-left: string[] [] -> [w720]
          shift-right: [w722] -> w703
          shift-left: w706 -> [w717]
          tunnel: w702 -> [w718] mode=indexing
          n202 = Search 1D Array(1D array=w717, element=w721) -> (index of element=w723:i32)  [unwired: 1 out]
          n203 = case shown="-1" w723 {
            tunnel: w717 -> [w725 w731]
            tunnel: [w725 w730] -> w722
            tunnel: w721 -> [_ w729]
            tunnel: w720 -> [w724 w728]
            tunnel: [w724 w727] -> w719
            tunnel: w718 -> [_ w726]
            frame 0, Default {
            }
            frame -1 {
              n204 = Build Array (concatenate)(w731, w729) -> (w730:string[])
              n205 = Build Array (concatenate)(w728, w726) -> (w727:string[])
            }
          }
        }
        n206 = for {
          tunnel: w701 -> [w714] mode=indexing
          tunnel: w700 -> [w716]
          tunnel: [w715] -> w699 mode=indexing
          n207 = Build Array (concatenate)(w714, w716) -> (w715:string[])
        }
      }
    }
    "Case" <- w39
  }
  "Filetype" <- w14
  "Results file Out" <- w12
  "Ch names Out" <- w11
  "Channel Values Out" <- w10
  "String Before" <- w9
  "String After" <- w7
  "Template File Out" <- w6
  "EOF?" <- w4
  "mark after read (chars.)" <- w3
  "Row numbers" <- w2
